vi "finction.vi"() -> ()   [LabVIEW 2017]
panel:
  out "f(x)":dbl
  in  "x":dbl
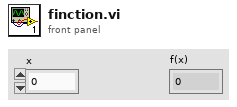
[diagram p1: front panel]
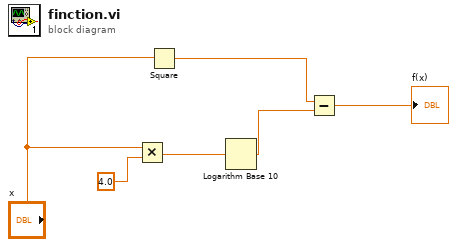
[diagram p0: block diagram]
diagram:
  n1 = Multiply(x="x", y=4.0) -> (x*y=w4:dbl)
  n2 = Square(x="x") -> (x^2=w3:dbl)
  n3 = Logarithm Base 10(1:w4) -> (0:w2:dbl)
  n4 = Subtract(x=w3, y=w2) -> (x-y=→"f(x)":dbl)
